vi "Time.vi"(8 "error in (no error)":errorcluster, 10 "Control In":T1={"I-O.lvclass"=refnum, "Gantry"=refnum, "Dispenser"="COM1"}, 11 "Sensor Dispense in":refnum<class "Sensor Dispense.lvclass">) -> (0 "error out":errorcluster, 1 "Timing Data":i32[](array[numeric]), 2 "Control Out":T1={"I-O.lvclass"=refnum, "Gantry"=refnum, "Dispenser"="COM1"}, 3 "Sensor Dispense out":refnum<class "Sensor Dispense.lvclass">)   [LabVIEW 2021, in "Sensor Dispense.lvclass"]
uses:
  Projects/Sensor Dispense.lvclass
  C:/Users/hep/Documents/UCSB-CMU-GantryCode/UCSB-Gantry-HEP-main (3)/UCSB-Gantry-HEP-main/Classes/Routine/Dispense/Dispense.lvclass
  Controller/Controllers.ctl
  Controller/I-O/I-O.lvclass
  C:/Program Files (x86)/Aerotech/A3200/LabVIEW/2010/Bin/Aerotech.A3200.dll
  Program Files (x86)/Aerotech/A3200/LabVIEW/2010/Bin/Aerotech.A3200.dll
  Projects/Sensor Dispense.lvclass/Sensor Dispense.ctl
  Controller/Motion/Motion.lvclass
  Controller/Motion/A3200/A3200.lvclass
  Controller/Controller.lvclass
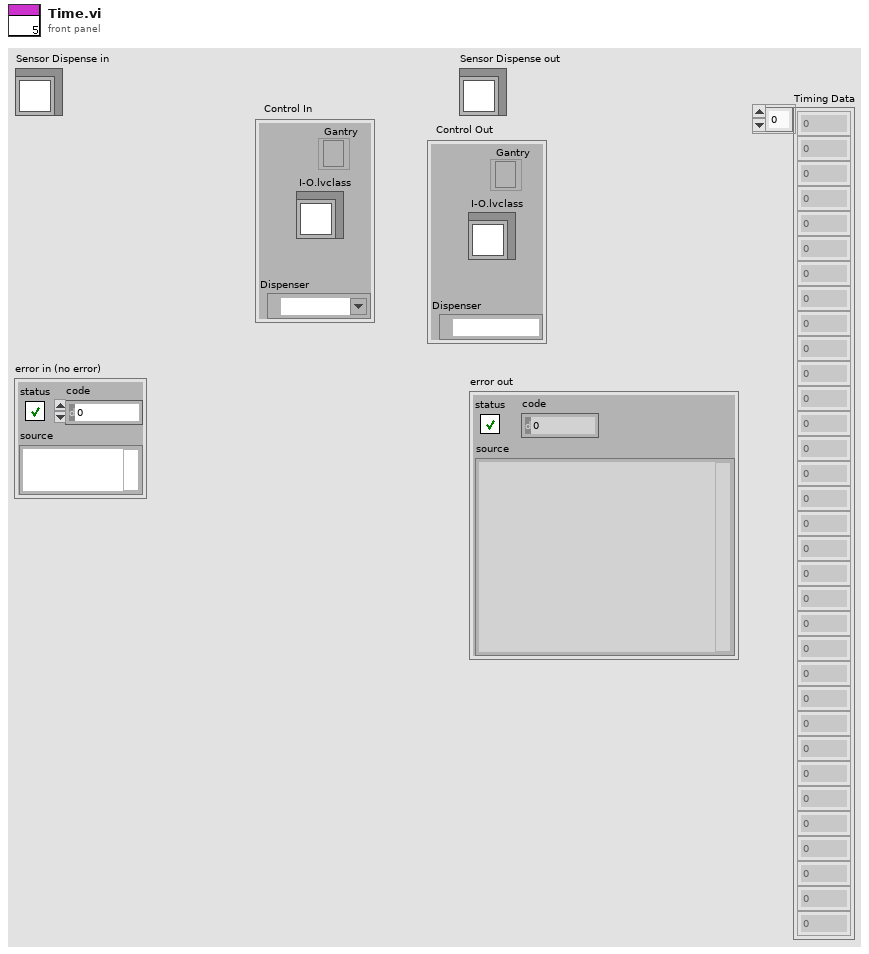
[diagram p1: front panel]
types:
  T1 = typedef "Controller.lvclass/Controllers.ctl" = cluster{"I-O.lvclass":refnum<class "I-O.lvclass">, "Gantry":refnum<k24>, "Dispenser":refnum<visa-resource-name>}
  T2 = cluster{"Endpoints":dbl[][], "Center":dbl[], "CW/CCW":dbl, "Dispense Type":enum16{"N-gon", "Square", "Arc", "Dot", "Line", "Circle"}}[]
  T3 = cluster{"Endpoints":dbl[][], "Center":dbl[], "CW/CCW":dbl, "Dispense Type":enum16{"N-gon", "Square", "Arc", "Dot", "Line", "Circle"}}
  T4 = enum16{"N-gon", "Square", "Arc", "Dot", "Line", "Circle"}
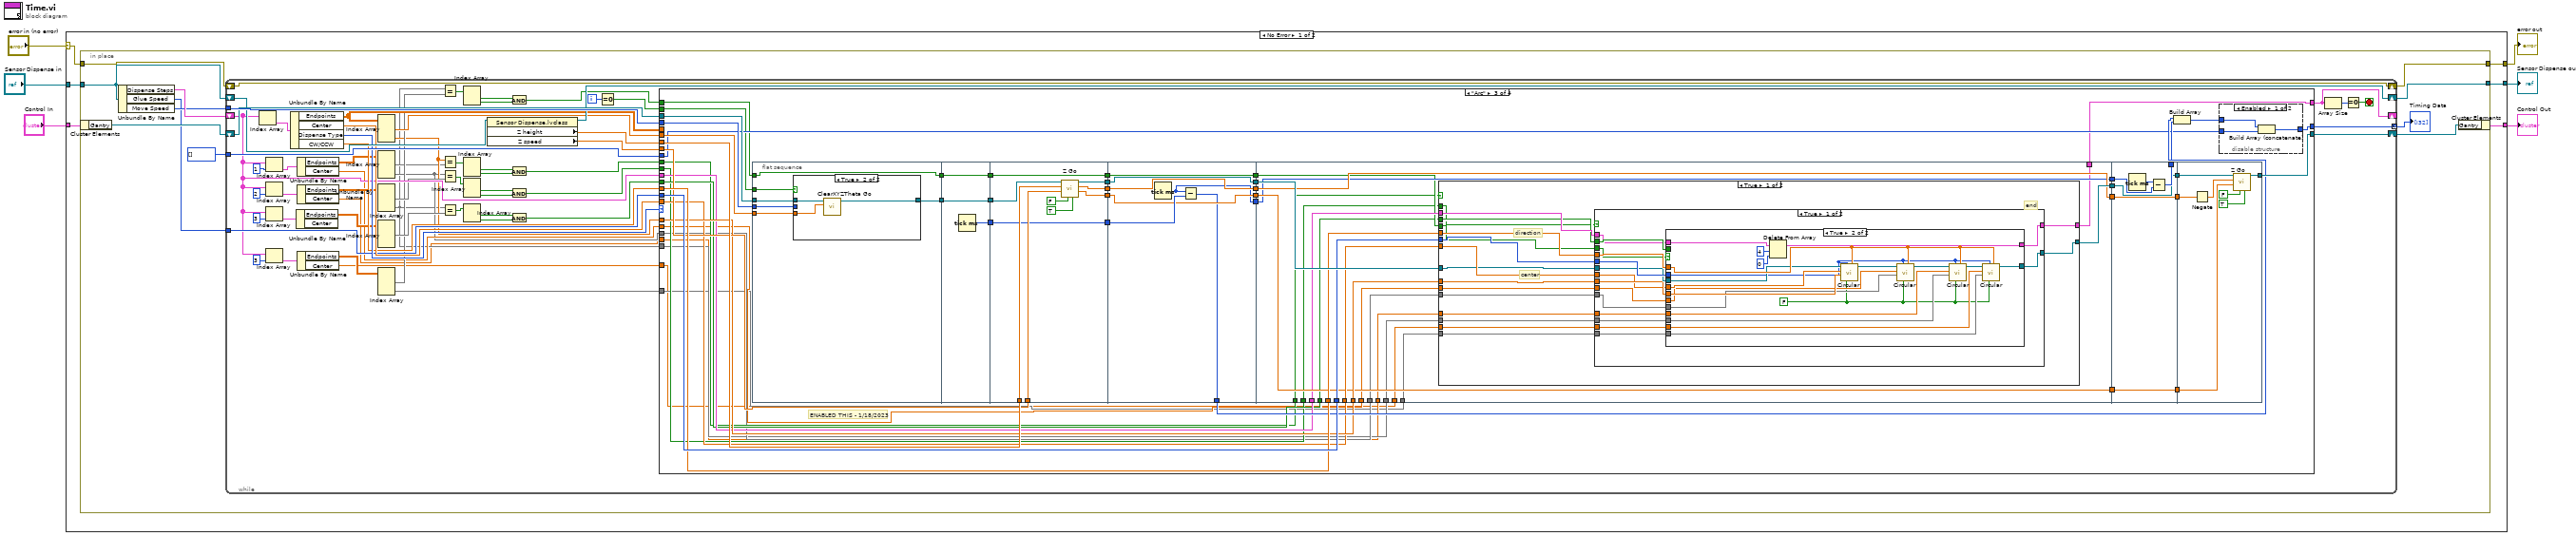
[diagram p0: block diagram]
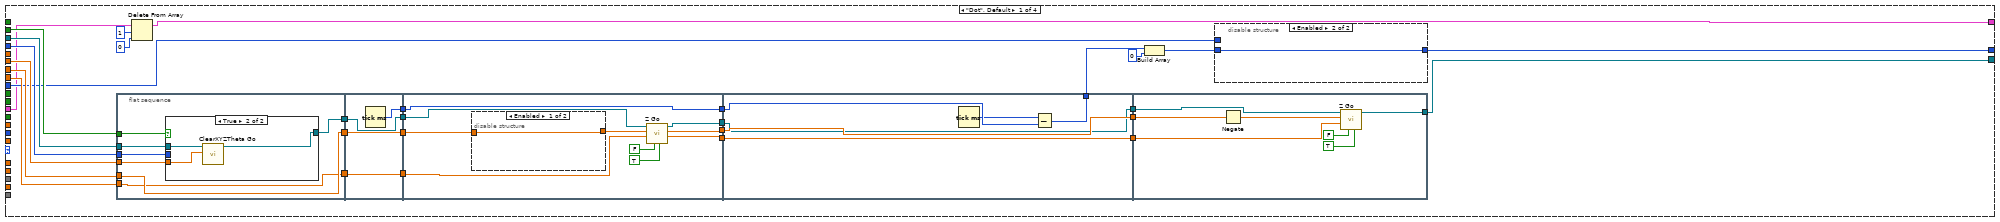
[diagram p2: hidden frame]
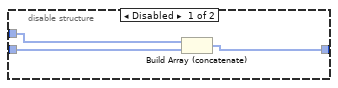
[diagram p3: hidden frame]
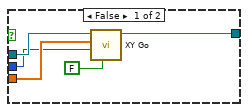
[diagram p4: hidden frame]
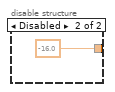
[diagram p5: hidden frame]
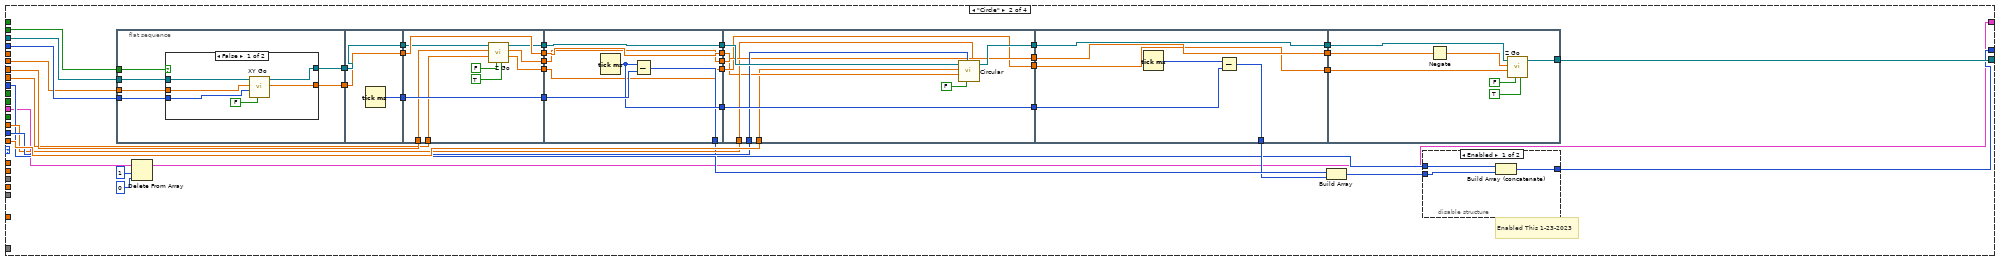
[diagram p6: hidden frame]
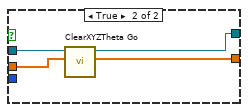
[diagram p8: hidden frame]
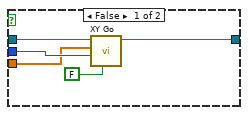
[diagram p10: hidden frame]
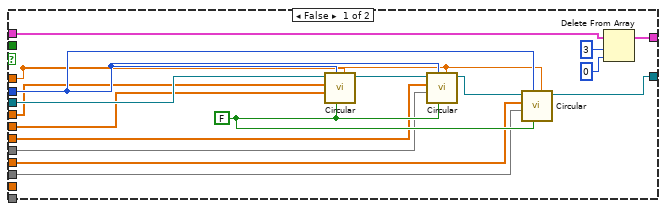
[diagram p11: hidden frame]
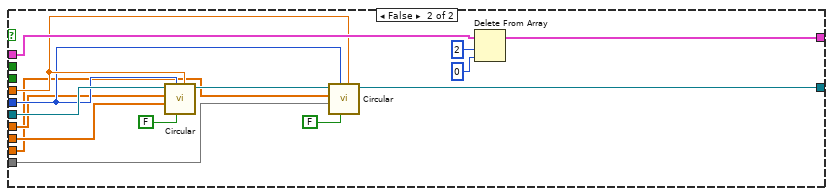
[diagram p12: hidden frame]
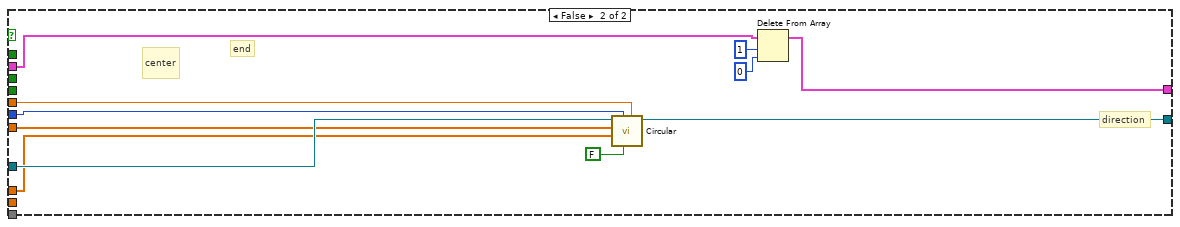
[diagram p13: hidden frame]
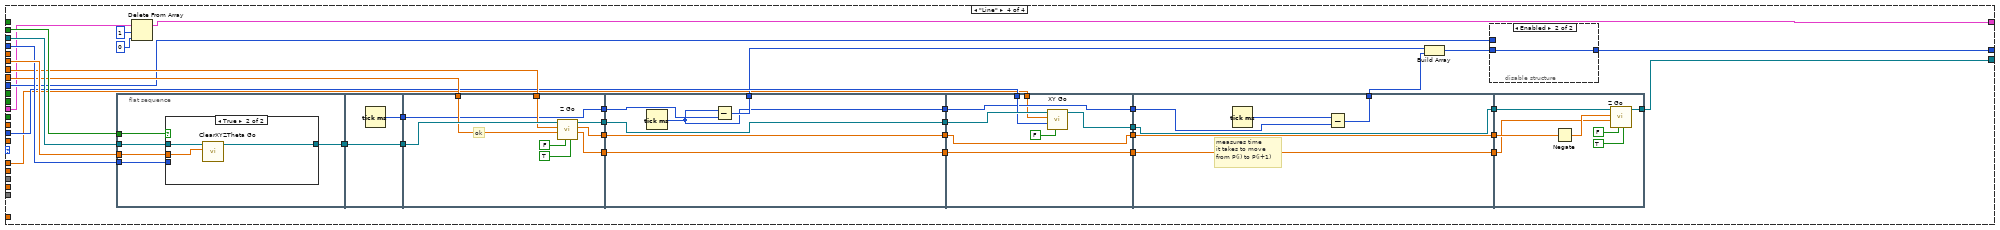
[diagram p14: hidden frame]
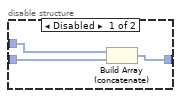
[diagram p15: hidden frame]
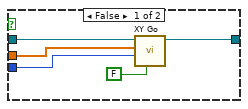
[diagram p16: hidden frame]
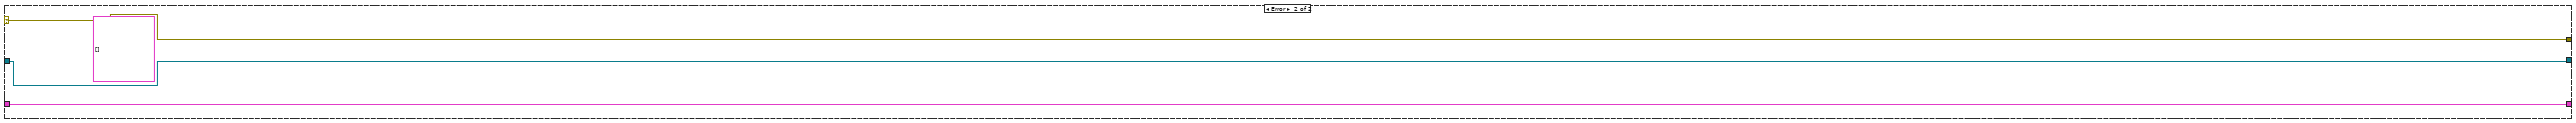
[diagram p17: hidden frame]
diagram:
  n1 = case shown="No Error" "error in (no error)" {
    selector: "error in (no error)" -> [w7 w579]
    tunnel: "Sensor Dispense in" -> [w12 w577]
    tunnel: [w11 w577] -> w5
    tunnel: "Control In" -> [w10 w578]
    tunnel: [w9 w578] -> w3
    tunnel: [w8 w579] -> w2
    frame No Error {
      n2 = in-place {
        in-place-border: w12 -> [w21]
        in-place-border: [w20] -> w11
        in-place-border: [w16] -> w8
        in-place-border: w7 -> [w15]
        n3 = in-place-cluster #1(w10) -> ("Gantry"=w22:refnum<k24>)
        n4 = Unbundle By Name "Unbundle By Name"(w21) -> ("Dispense Steps"=w17:T2, "Glue Speed"=w13:i32, "Move Speed"=w14:i32)
        n5 = while {
          tunnel: w14 -> [w85]
          shift-right: [w73] -> w19
          shift-left: w22 -> [w83]
          tunnel: w13 -> [w70]
          shift-right: [w81] -> w20
          shift-left: w21 -> [w82]
          shift-right: [w25] -> w16
          shift-left: w15 -> [w25]
          tunnel: i32[] [] -> [w84]
          tunnel: [w76] -> w18 mode=concatenating
          shift-right: [w27] -> _
          shift-left: w17 -> [w62]
          i -> [w80]
          stop <- w24 stop-if-true
          n6 = Index Array(array=w62) -> (element=w66:T3)  [unwired: 1 in]
          n7 = Index Array(array=w62, index=1) -> (element=w63:T3)
          n8 = Index Array(array=w62, index=2) -> (element=w64:T3)
          n9 = Index Array(array=w62, index=3) -> (element=w65:T3)
          n10 = Index Array(array=w62, index=3) -> (element=w68:T3)
          n11 = Unbundle By Name(w66) -> ("Endpoints"=w72:dbl[][], "Center"=w71:dbl[], "Dispense Type"=w75:T4, "CW/CCW"=w69:dbl)
          n12 = Unbundle By Name(w65) -> ("Endpoints"=w56:dbl[][])  [unwired: 1 out]
          n13 = Unbundle By Name(w63) -> ("Endpoints"=w55:dbl[][], "Center"=w33:dbl[])
          n14 = Unbundle By Name(w64) -> ("Endpoints"=w57:dbl[][], "Center"=w30:dbl[])
          n15 = Unbundle By Name(w68) -> ("Endpoints"=w58:dbl[][], "Center"=w28:dbl[])
          n16 = Index Array(array=w72) -> (element #1=w74:dbl[], element #2=w37:dbl[])  [unwired: 4 in]
          n17 = Index Array(array=w55) -> (element #1=w36:dbl[], element #2=w32:dbl[])  [unwired: 4 in]
          n18 = Index Array(array=w57) -> (element #1=w45:dbl[], element #2=w31:dbl[])  [unwired: 4 in]
          n19 = Index Array(array=w56) -> (element #1=w50:dbl[])  [unwired: 4 in, 1 out]
          n20 = Index Array(array=w58) -> (element #1=w38:dbl[], element #2=w29:dbl[])  [unwired: 4 in]
          n21 = Equal?(x=w31, y=w38) -> (x = y?=w54:bool[])
          n22 = Equal?(x=w37, y=w36) -> (x = y?=w41:bool[])
          n23 = Equal?(x=w32, y=w45) -> (x = y?=w44:bool[])
          n24 = Equal?(x=w31, y=w50) -> (x = y?=w49:bool[])
          n25 = Index Array(array=w54) -> (element #1=w53:bool, element #2=w52:bool)  [unwired: 2 in]
          n26 = Index Array(array=w41) -> (element #1=w40:bool, element #2=w39:bool)  [unwired: 2 in]
          n27 = Index Array(array=w44) -> (element #1=w43:bool, element #2=w42:bool)  [unwired: 2 in]
          n28 = Index Array(array=w49) -> (element #1=w48:bool, element #2=w47:bool)  [unwired: 2 in]
          n29 = property class="Sensor Dispense.lvclass"(reference=w82) -> (reference out=w81:refnum<class "Sensor Dispense.lvclass">, "Z height"=w78:dbl, "Z speed"=w77:dbl)  [unwired: 1 in, 1 out]
          n30 = And(x=w53, y=w52) -> (x .and. y?=w51:bool)
          n31 = And(x=w40, y=w39) -> (x .and. y?=w34:bool)
          n32 = And(x=w43, y=w42) -> (x .and. y?=w35:bool)
          n33 = And(x=w48, y=w47) -> (x .and. y?=w46:bool)
          n34 = Equal To 0?(x=w80) -> (x = 0?=w79:bool)
          n35 = case shown="\"Arc\"" w75 {
            tunnel: w71 -> [_ w192 w292 _]
            tunnel: w83 -> [w111 w193 w317 w521]
            tunnel: w85 -> [w95 w181 w315 w519]
            tunnel: [w96 w200 w304 w495] -> w73
            tunnel: w70 -> [_ w191 w314 w509]
            tunnel: w69 -> [_ w190 w313 _]
            tunnel: w84 -> [w92 w187 w296 w493]
            tunnel: [w90 w185 w295 w491] -> w76
            tunnel: w74 -> [w112 w180 w316 w520]
            tunnel: w77 -> [w105 w183 w311 w514]
            tunnel: w78 -> [w108 w184 w312 w515]
            tunnel: w79 -> [w113 w182 w294 w518]
            tunnel: w72 -> [_ _ _ _]
            tunnel: w37 -> [_ _ w293 w490]
            tunnel: w62 -> [w89 w167 w283 w487]
            tunnel: [w88 w166 w282 w486] -> w27
            tunnel: w51 -> [_ _ w277 _]
            tunnel: w46 -> [_ _ w276 _]
            tunnel: w35 -> [_ _ w275 _]
            tunnel: w34 -> [_ _ w274 _]
            tunnel: w33 -> [_ _ w273 _]
            tunnel: w32 -> [_ _ w272 _]
            tunnel: w31 -> [_ _ w271 _]
            tunnel: w30 -> [_ _ w270 _]
            tunnel: w29 -> [_ _ w269 _]
            tunnel: w28 -> [_ _ w268 _]
            frame "Dot", Default {
              n36 = flat-sequence {
                tunnel: w113 -> [w126]
                tunnel: w112 -> [w125]
                tunnel: w111 -> [w124]
                tunnel: [w123] -> w109
                tunnel: w108 -> [w122]
                tunnel: [w122] -> w106
                tunnel: w105 -> [w121]
                tunnel: [w121] -> w103
                tunnel: w95 -> [w120]
                tunnel: [w138] -> w115
                tunnel: [w137] -> w110
                tunnel: w109 -> [w137]
                tunnel: [w136] -> w107
                tunnel: w106 -> [w136]
                tunnel: [w135] -> w104
                tunnel: w103 -> [w135]
                tunnel: [w148] -> w114
                tunnel: w115 -> [w148]
                tunnel: w110 -> [w147]
                tunnel: w107 -> [w140]
                tunnel: w104 -> [w146]
                tunnel: [w145] -> w101
                tunnel: [w144] -> w99
                tunnel: [w143] -> w97
                tunnel: w114 -> [w156]
                tunnel: [w154] -> w94
                tunnel: [w153] -> w102
                tunnel: w101 -> [w153]
                tunnel: [w152] -> w100
                tunnel: w99 -> [w152]
                tunnel: [w151] -> w98
                tunnel: w97 -> [w151]
                tunnel: w102 -> [w163]
                tunnel: w100 -> [w161]
                tunnel: w98 -> [w160]
                tunnel: [w159] -> w96
                frame #0 {
                  n37 = case shown="True" w126 {
                    tunnel: w125 -> [w129 w134]
                    tunnel: w124 -> [w131 w133]
                    tunnel: [w130 w132] -> w123
                    tunnel: w120 -> [w128 _]
                    frame False {
                      n38 = call "XY Go.vi"("return immediately"=FALSE, "Speed"=w128, "XY In"=w129, "Gantry In"=w131) -> ("Gantry Out"=w130:refnum<k24>)  [unwired: 5 in, 2 out]
                    }
                    frame True {
                      n39 = call "ClearXYZTheta Go.vi"("XYZTheta In"=w134, "Gantry In"=w133) -> ("Gantry Out"=w132:refnum<k24>)  [unwired: 7 in, 2 out]
                    }
                  }
                }
                frame #1 {
                  n40 = Tick Count (ms)() -> (millisecond timer value=w138:u32)
                }
                frame #2 {
                  n41 = disable-structure shown="Enabled" {
                    disable-tunnel: w140 -> [w149 _]
                    disable-tunnel: [w149 -16.0 ("Z height")] -> w139
                    frame Enabled {
                    }
                    frame Disabled {
                    }
                  }
                  n42 = call "Z Go.vi"("Increment"=TRUE, "Return Immediately"=FALSE, "Speed In"=w146, "Position In"=w139, "Gantry In"=w147) -> ("Speed Out"=w144:dbl, "Position Out"=w145:dbl, "Gantry Out"=w143:refnum<k24>)  [unwired: 3 in, 1 out]
                }
                frame #3 {
                  n43 = Tick Count (ms)() -> (millisecond timer value=w155:u32)
                  n44 = Subtract(x=w155, y=w156) -> (x-y=w154:u32)
                }
                frame #4 {
                  n45 = Negate(x=w163) -> (-x=w162:dbl)
                  n46 = call "Z Go.vi"("Increment"=TRUE, "Return Immediately"=FALSE, "Speed In"=w161, "Position In"=w162, "Gantry In"=w160) -> ("Gantry Out"=w159:refnum<k24>)  [unwired: 3 in, 3 out]
                }
              }
              n47 = Delete From Array(array=w89, length=1, index=0) -> (array with subset deleted=w88:T2)  [unwired: 1 out]
              n48 = Build Array(w94, u32 0 ("element")) -> (w91:u32[])
              n49 = disable-structure shown="Enabled" {
                disable-tunnel: w92 -> [w118 _]
                disable-tunnel: w91 -> [w117 w119]
                disable-tunnel: [w116 w119] -> w90
                frame Disabled {
                  n50 = Build Array (concatenate)(w118, w117) -> (w116:u32[])
                }
                frame Enabled {
                }
              }
            }
            frame "Circle" {
              # "Enabled This 1-23-2023"
              n51 = flat-sequence {
                tunnel: [w211] -> w198
                tunnel: w193 -> [w212]
                tunnel: w180 -> [w213]
                tunnel: w182 -> [w214]
                tunnel: w181 -> [w210]
                tunnel: [w209] -> w176
                tunnel: [w227] -> w204
                tunnel: [w226] -> w199
                tunnel: w198 -> [w226]
                tunnel: [w225] -> w177
                tunnel: w176 -> [w225]
                tunnel: w204 -> [w237]
                tunnel: [w237] -> w203
                tunnel: w199 -> [w235]
                tunnel: [w234] -> w197
                tunnel: w184 -> [w233]
                tunnel: w183 -> [w232]
                tunnel: [w236] -> w178
                tunnel: w177 -> [w236]
                tunnel: [w231] -> w173
                tunnel: [w230] -> w170
                tunnel: w203 -> [w244]
                tunnel: [w243] -> w201
                tunnel: [w242] -> w189
                tunnel: w197 -> [w241]
                tunnel: [w241] -> w196
                tunnel: [w240] -> w179
                tunnel: w178 -> [w240]
                tunnel: [w239] -> w174
                tunnel: w173 -> [w239]
                tunnel: [w238] -> w171
                tunnel: w170 -> [w238]
                tunnel: [w254] -> w202
                tunnel: w201 -> [w254]
                tunnel: w196 -> [w253]
                tunnel: [w252] -> w194
                tunnel: w192 -> [w246]
                tunnel: w191 -> [w251]
                tunnel: w190 -> [w248]
                tunnel: w179 -> [w247]
                tunnel: [w250] -> w175
                tunnel: w174 -> [w250]
                tunnel: [w249] -> w172
                tunnel: w171 -> [w249]
                tunnel: w202 -> [w259]
                tunnel: [w258] -> w188
                tunnel: [w257] -> w195
                tunnel: w194 -> [w257]
                tunnel: w175 -> [w256]
                tunnel: w172 -> [w255]
                tunnel: [w256] -> w169
                tunnel: [w255] -> w168
                tunnel: [w265] -> w200
                tunnel: w195 -> [w266]
                tunnel: w169 -> [w267]
                tunnel: w168 -> [w264]
                frame #0 {
                  n52 = case shown="False" w214 {
                    tunnel: w213 -> [w215 w222]
                    tunnel: w212 -> [w220 w224]
                    tunnel: [w219 w223] -> w211
                    tunnel: w210 -> [w218 _]
                    tunnel: [w217 w221] -> w209
                    frame False {
                      n53 = call "XY Go.vi"("return immediately"=FALSE, "Speed"=w218, "XY In"=w215, "Gantry In"=w220) -> ("XY Out"=w217:dbl[], "Gantry Out"=w219:refnum<k24>)  [unwired: 5 in, 1 out]
                    }
                    frame True {
                      n54 = call "ClearXYZTheta Go.vi"("XYZTheta In"=w222, "Gantry In"=w224) -> ("XYZTheta Out"=w221:dbl[], "Gantry Out"=w223:refnum<k24>)  [unwired: 7 in, 1 out]
                    }
                  }
                }
                frame #1 {
                  n55 = Tick Count (ms)() -> (millisecond timer value=w227:u32)
                }
                frame #2 {
                  n56 = call "Z Go.vi"("Increment"=TRUE, "Return Immediately"=FALSE, "Speed In"=w232, "Position In"=w233, "Gantry In"=w235) -> ("Speed Out"=w230:dbl, "Position Out"=w231:dbl, "Gantry Out"=w234:refnum<k24>)  [unwired: 3 in, 1 out]
                }
                frame #3 {
                  n57 = Tick Count (ms)() -> (millisecond timer value=w243:u32)
                  n58 = Subtract(x=w243, y=w244) -> (x-y=w242:u32)
                }
                frame #4 {
                  n59 = call "Circular.vi"("Direction"=w248, "return immediately"=FALSE, "Speed"=w251, "XY End"=w247, "XY Center"=w246, "Gantry In"=w253) -> ("Gantry Out"=w252:refnum<k24>)  [unwired: 4 in, 1 out]
                }
                frame #5 {
                  n60 = Tick Count (ms)() -> (millisecond timer value=w260:u32)
                  n61 = Subtract(x=w260, y=w259) -> (x-y=w258:u32)
                }
                frame #6 {
                  n62 = Negate(x=w267) -> (-x=w263:dbl)
                  n63 = call "Z Go.vi"("Increment"=TRUE, "Return Immediately"=FALSE, "Speed In"=w264, "Position In"=w263, "Gantry In"=w266) -> ("Gantry Out"=w265:refnum<k24>)  [unwired: 3 in, 3 out]
                }
              }
              n64 = Delete From Array(array=w167, length=1, index=0) -> (array with subset deleted=w166:T2)  [unwired: 1 out]
              n65 = Build Array(w189, w188) -> (w186:u32[])
              n66 = disable-structure shown="Enabled" {
                disable-tunnel: w187 -> [w207 _]
                disable-tunnel: w186 -> [w206 w208]
                disable-tunnel: [w205 w208] -> w185
                frame Enabled {
                  n67 = Build Array (concatenate)(w207, w206) -> (w205:u32[])
                }
                frame Disabled {
                }
              }
            }
            frame "Arc" {
              # "ENABLED THIS - 1/18/2023"
              n68 = flat-sequence {
                tunnel: w317 -> [w327]
                tunnel: w316 -> [w326]
                tunnel: w315 -> [w325]
                tunnel: [w324] -> w308
                tunnel: w294 -> [w323]
                tunnel: [w322] -> w278
                tunnel: w277 -> [w322]
                tunnel: w308 -> [w338]
                tunnel: [w338] -> w307
                tunnel: [w337] -> w305
                tunnel: [w336] -> w279
                tunnel: w278 -> [w336]
                tunnel: w307 -> [w348]
                tunnel: [w345] -> w310
                tunnel: w312 -> [w347]
                tunnel: w311 -> [w346]
                tunnel: [w344] -> w306
                tunnel: w305 -> [w344]
                tunnel: [w343] -> w302
                tunnel: [w342] -> w300
                tunnel: [w339] -> w280
                tunnel: w279 -> [w339]
                tunnel: w310 -> [w355]
                tunnel: [w355] -> w309
                tunnel: w306 -> [w354]
                tunnel: [w353] -> w303
                tunnel: w302 -> [w353]
                tunnel: [w352] -> w301
                tunnel: w300 -> [w352]
                tunnel: [w351] -> w299
                tunnel: [w350] -> w285
                tunnel: [w349] -> w281
                tunnel: w280 -> [w349]
                tunnel: w309 -> [w376]
                tunnel: w314 -> [w375]
                tunnel: w313 -> [w374]
                tunnel: w303 -> [w370]
                tunnel: w301 -> [w369]
                tunnel: w292 -> [w373]
                tunnel: w293 -> [w372]
                tunnel: [w371] -> w290
                tunnel: [w370] -> w288
                tunnel: [w369] -> w286
                tunnel: w285 -> [w368]
                tunnel: [w368] -> w284
                tunnel: w283 -> [w367]
                tunnel: [w366] -> w282
                tunnel: w281 -> [w365]
                tunnel: w276 -> [w364]
                tunnel: w275 -> [w362]
                tunnel: w274 -> [w363]
                tunnel: w273 -> [w361]
                tunnel: w272 -> [w360]
                tunnel: w271 -> [w359]
                tunnel: w270 -> [w358]
                tunnel: w269 -> [w357]
                tunnel: w268 -> [w356]
                tunnel: [w478] -> w298
                tunnel: [w477] -> w291
                tunnel: w290 -> [w477]
                tunnel: [w476] -> w289
                tunnel: w288 -> [w476]
                tunnel: [w475] -> w287
                tunnel: w286 -> [w475]
                tunnel: w284 -> [w473]
                tunnel: [w485] -> w304
                tunnel: w291 -> [w483]
                tunnel: w289 -> [w482]
                tunnel: w287 -> [w481]
                frame #0 {
                  n69 = case shown="True" w323 {
                    tunnel: [w332 w335] -> w324
                    tunnel: w327 -> [w331 w334]
                    tunnel: w326 -> [w328 w333]
                    tunnel: w325 -> [w330 _]
                    frame False {
                      n70 = call "XY Go.vi"("return immediately"=FALSE, "Speed"=w330, "XY In"=w328, "Gantry In"=w331) -> ("Gantry Out"=w332:refnum<k24>)  [unwired: 5 in, 2 out]
                    }
                    frame True {
                      n71 = call "ClearXYZTheta Go.vi"("XYZTheta In"=w333, "Gantry In"=w334) -> ("Gantry Out"=w335:refnum<k24>)  [unwired: 7 in, 2 out]
                    }
                  }
                }
                frame #1 {
                  n72 = Tick Count (ms)() -> (millisecond timer value=w337:u32)
                }
                frame #2 {
                  n73 = call "Z Go.vi"("Increment"=TRUE, "Return Immediately"=FALSE, "Speed In"=w346, "Position In"=w347, "Gantry In"=w348) -> ("Speed Out"=w342:dbl, "Position Out"=w343:dbl, "Gantry Out"=w345:refnum<k24>)  [unwired: 3 in, 1 out]
                }
                frame #3 {
                  n74 = Tick Count (ms)() -> (millisecond timer value=w350:u32)
                  n75 = Subtract(x=w350, y=w354) -> (x-y=w351:u32)
                }
                frame #4 {
                  n76 = case shown="True" w363 {
                    tunnel: w376 -> [w388 w472]
                    tunnel: w375 -> [w386 w471]
                    tunnel: w374 -> [w391 w470]
                    tunnel: w373 -> [w390 w469]
                    tunnel: w372 -> [w389 w468]
                    tunnel: [w387 w467] -> w371
                    tunnel: w367 -> [w393 w463]
                    tunnel: [w392 w462] -> w366
                    tunnel: w365 -> [w385 _]
                    tunnel: w364 -> [w384 _]
                    tunnel: w362 -> [w383 _]
                    tunnel: w361 -> [w382 _]
                    tunnel: w360 -> [w381 _]
                    tunnel: w359 -> [w380 _]
                    tunnel: w358 -> [w379 _]
                    tunnel: w357 -> [w378 _]
                    tunnel: w356 -> [w377 _]
                    frame True {
                      # "direction"
                      # "center"
                      # "end"
                      n77 = case shown="True" w383 {
                        tunnel: w393 -> [w395 w461]
                        tunnel: [w394 w458] -> w392
                        tunnel: w391 -> [w409 w457]
                        tunnel: w390 -> [w404 w450]
                        tunnel: w389 -> [w405 w449]
                        tunnel: w388 -> [w407 w456]
                        tunnel: [w406 w454] -> w387
                        tunnel: w386 -> [w408 w453]
                        tunnel: w385 -> [w403 _]
                        tunnel: w384 -> [w402 _]
                        tunnel: w382 -> [w401 w448]
                        tunnel: w381 -> [w400 w447]
                        tunnel: w380 -> [w399 _]
                        tunnel: w379 -> [w398 _]
                        tunnel: w378 -> [w397 _]
                        tunnel: w377 -> [w396 _]
                        frame True {
                          n78 = case shown="True" w403 {
                            tunnel: w409 -> [w421 w446]
                            tunnel: w408 -> [w422 w431]
                            tunnel: w407 -> [w426 w439]
                            tunnel: [w423 w435] -> w406
                            tunnel: w405 -> [w420 w444]
                            tunnel: w404 -> [w419 w445]
                            tunnel: w402 -> [_ _]
                            tunnel: w401 -> [w417 w442]
                            tunnel: w400 -> [w416 w443]
                            tunnel: w399 -> [w415 w441]
                            tunnel: w398 -> [w414 w440]
                            tunnel: w397 -> [_ w434]
                            tunnel: w396 -> [_ w433]
                            tunnel: w395 -> [w411 w430]
                            tunnel: [w410 w429] -> w394
                            frame False {
                              w418 = FALSE
                              n79 = call "Circular.vi"("Direction"=w421, "return immediately"=w418, "Speed"=w422, "XY End"=w420, "XY Center"=w419, "Gantry In"=w426) -> ("Gantry Out"=w425:refnum<k24>)  [unwired: 4 in, 1 out]
                              n80 = call "Circular.vi"("Direction"=w421, "return immediately"=w418, "Speed"=w422, "XY End"=w416, "XY Center"=w417, "Gantry In"=w425) -> ("Gantry Out"=w424:refnum<k24>)  [unwired: 4 in, 1 out]
                              n81 = call "Circular.vi"("Direction"=w421, "return immediately"=w418, "Speed"=w422, "XY End"=w415, "XY Center"=w414, "Gantry In"=w424) -> ("Gantry Out"=w423:refnum<k24>)  [unwired: 4 in, 1 out]
                              n82 = Delete From Array(array=w411, length=3, index=0) -> (array with subset deleted=w410:T2)  [unwired: 1 out]
                            }
                            frame True {
                              w432 = FALSE
                              n83 = Delete From Array(array=w430, length=4, index=0) -> (array with subset deleted=w429:T2)  [unwired: 1 out]
                              n84 = call "Circular.vi"("Direction"=w446, "return immediately"=w432, "Speed"=w431, "XY End"=w444, "XY Center"=w445, "Gantry In"=w439) -> ("Gantry Out"=w438:refnum<k24>)  [unwired: 4 in, 1 out]
                              n85 = call "Circular.vi"("Direction"=w446, "return immediately"=w432, "Speed"=w431, "XY End"=w443, "XY Center"=w442, "Gantry In"=w438) -> ("Gantry Out"=w437:refnum<k24>)  [unwired: 4 in, 1 out]
                              n86 = call "Circular.vi"("Direction"=w446, "return immediately"=w432, "Speed"=w431, "XY End"=w441, "XY Center"=w440, "Gantry In"=w437) -> ("Gantry Out"=w436:refnum<k24>)  [unwired: 4 in, 1 out]
                              n87 = call "Circular.vi"("Direction"=w446, "return immediately"=w432, "Speed"=w431, "XY End"=w434, "XY Center"=w433, "Gantry In"=w436) -> ("Gantry Out"=w435:refnum<k24>)  [unwired: 4 in, 1 out]
                            }
                          }
                        }
                        frame False {
                          n88 = call "Circular.vi"("Direction"=w457, "return immediately"=FALSE, "Speed"=w453, "XY End"=w449, "XY Center"=w450, "Gantry In"=w456) -> ("Gantry Out"=w455:refnum<k24>)  [unwired: 4 in, 1 out]
                          n89 = call "Circular.vi"("Direction"=w457, "return immediately"=FALSE, "Speed"=w453, "XY End"=w447, "XY Center"=w448, "Gantry In"=w455) -> ("Gantry Out"=w454:refnum<k24>)  [unwired: 4 in, 1 out]
                          n90 = Delete From Array(array=w461, length=2, index=0) -> (array with subset deleted=w458:T2)  [unwired: 1 out]
                        }
                      }
                    }
                    frame False {
                      # "end"
                      # "center"
                      # "direction"
                      n91 = call "Circular.vi"("Direction"=w470, "return immediately"=FALSE, "Speed"=w471, "XY End"=w468, "XY Center"=w469, "Gantry In"=w472) -> ("Gantry Out"=w467:refnum<k24>)  [unwired: 4 in, 1 out]
                      n92 = Delete From Array(array=w463, length=1, index=0) -> (array with subset deleted=w462:T2)  [unwired: 1 out]
                    }
                  }
                }
                frame #5 {
                  n93 = Tick Count (ms)() -> (millisecond timer value=w474:u32)
                  n94 = Subtract(x=w474, y=w473) -> (x-y=w478:u32)
                }
                frame #6 {
                  n95 = Negate(x=w482) -> (-x=w484:dbl)
                  n96 = call "Z Go.vi"("Increment"=TRUE, "Return Immediately"=FALSE, "Speed In"=w481, "Position In"=w484, "Gantry In"=w483) -> ("Gantry Out"=w485:refnum<k24>)  [unwired: 3 in, 3 out]
                }
              }
              n97 = Build Array "Build Array"(w299, w298) -> (w297:u32[])
              n98 = disable-structure shown="Enabled" {
                disable-tunnel: w297 -> [w320 w321]
                disable-tunnel: w296 -> [w319 _]
                disable-tunnel: [w318 w321] -> w295
                frame Enabled {
                  n99 = Build Array (concatenate) "Build Array"(w320, w319) -> (w318:u32[])
                }
                frame Disabled {
                }
              }
            }
            frame "Line" {
              n100 = flat-sequence {
                tunnel: w521 -> [w530]
                tunnel: w520 -> [w526]
                tunnel: w519 -> [w529]
                tunnel: w518 -> [w528]
                tunnel: [w527] -> w517
                tunnel: w517 -> [w539]
                tunnel: [w539] -> w516
                tunnel: [w540] -> w512
                tunnel: w516 -> [w549]
                tunnel: w515 -> [w548]
                tunnel: w514 -> [w547]
                tunnel: [w546] -> w513
                tunnel: w512 -> [w546]
                tunnel: [w545] -> w510
                tunnel: [w544] -> w501
                tunnel: [w543] -> w497
                tunnel: w513 -> [w555]
                tunnel: [w554] -> w494
                tunnel: [w553] -> w511
                tunnel: w510 -> [w553]
                tunnel: [w552] -> w507
                tunnel: [w551] -> w502
                tunnel: w501 -> [w551]
                tunnel: [w550] -> w498
                tunnel: w497 -> [w550]
                tunnel: w511 -> [w563]
                tunnel: w509 -> [w562]
                tunnel: [w561] -> w508
                tunnel: w507 -> [w561]
                tunnel: [w560] -> w505
                tunnel: [w559] -> w503
                tunnel: w502 -> [w559]
                tunnel: [w558] -> w499
                tunnel: w498 -> [w558]
                tunnel: w490 -> [w557]
                tunnel: w508 -> [w568]
                tunnel: [w567] -> w496
                tunnel: [w566] -> w506
                tunnel: w505 -> [w566]
                tunnel: [w565] -> w504
                tunnel: w503 -> [w565]
                tunnel: [w564] -> w500
                tunnel: w499 -> [w564]
                tunnel: w506 -> [w576]
                tunnel: w504 -> [w575]
                tunnel: w500 -> [w573]
                tunnel: [w572] -> w495
                frame #0 {
                  n101 = case shown="True" w528 {
                    tunnel: w530 -> [w535 w538]
                    tunnel: w529 -> [w534 _]
                    tunnel: [w533 w537] -> w527
                    tunnel: w526 -> [w532 w536]
                    frame False {
                      n102 = call "XY Go.vi"("return immediately"=FALSE, "Speed"=w534, "XY In"=w532, "Gantry In"=w535) -> ("Gantry Out"=w533:refnum<k24>)  [unwired: 5 in, 2 out]
                    }
                    frame True {
                      n103 = call "ClearXYZTheta Go.vi"("XYZTheta In"=w536, "Gantry In"=w538) -> ("Gantry Out"=w537:refnum<k24>)  [unwired: 7 in, 2 out]
                    }
                  }
                }
                frame #1 {
                  n104 = Tick Count (ms)() -> (millisecond timer value=w540:u32)
                }
                frame #2 {
                  # "ok"
                  n105 = call "Z Go.vi"("Increment"=TRUE, "Return Immediately"=FALSE, "Speed In"=w547, "Position In"=w548, "Gantry In"=w549) -> ("Speed Out"=w543:dbl, "Position Out"=w544:dbl, "Gantry Out"=w545:refnum<k24>)  [unwired: 3 in, 1 out]
                }
                frame #3 {
                  n106 = Tick Count (ms)() -> (millisecond timer value=w552:u32)
                  n107 = Subtract(x=w552, y=w555) -> (x-y=w554:u32)
                }
                frame #4 {
                  n108 = call "XY Go.vi"("return immediately"=FALSE, "Speed"=w562, "XY In"=w557, "Gantry In"=w563) -> ("Gantry Out"=w560:refnum<k24>)  [unwired: 5 in, 2 out]
                }
                frame #5 {
                  # "measures time\nit takes to move\nfrom P(i) to P(i+1)"
                  n109 = Tick Count (ms)() -> (millisecond timer value=w569:u32)
                  n110 = Subtract(x=w569, y=w568) -> (x-y=w567:u32)
                }
                frame #6 {
                  n111 = Negate(x=w575) -> (-x=w574:dbl)
                  n112 = call "Z Go.vi"("Increment"=TRUE, "Return Immediately"=FALSE, "Speed In"=w573, "Position In"=w574, "Gantry In"=w576) -> ("Gantry Out"=w572:refnum<k24>)  [unwired: 3 in, 3 out]
                }
              }
              n113 = Delete From Array(array=w487, length=1, index=0) -> (array with subset deleted=w486:T2)  [unwired: 1 out]
              n114 = Build Array(w494, w496) -> (w492:u32[])
              n115 = disable-structure shown="Enabled" {
                disable-tunnel: w493 -> [w524 _]
                disable-tunnel: w492 -> [w523 w525]
                disable-tunnel: [w522 w525] -> w491
                frame Disabled {
                  n116 = Build Array (concatenate)(w524, w523) -> (w522:u32[])
                }
                frame Enabled {
                }
              }
            }
          }
          n117 = Array Size(array=w27) -> (size(s)=w26:i32)
          n118 = Equal To 0?(x=w26) -> (x = 0?=w24:bool)
        }
        "Timing Data" <- w18
        n119 = in-place-cluster #1("Gantry"=w19) -> (w9:T1)
      }
    }
    frame Error {
      (unwired) T2 [] ("Dispense Steps")
    }
  }
  "error out" <- w2
  "Sensor Dispense out" <- w5
  "Control Out" <- w3
